vi "Sub Super Duper_6_26a_PD.vi"(0 "VISA resource name":refnum<visa-resource-name>="GPIB0::17::INSTR", 1 "Sample Properties:":T5 {"Date Created" format="%<%Y/%m/%d>T"}, 2 "TRF Cluster":T6={"Step 4"=-38.0, "# of Loops"=1.0, "Transfer 2"=FALSE, "Start 4"=-2.0, "Total Points 2"=2, "Start 3"=40.0, "Stop 2"=-40.0, "Step 3"=-1.0, "Loop Step"=0.0, "Integration Time 3"=0, "Loop Wait"=0.0, "First Step"=0.0} {"Loop Wait" format="%<%H:%M:%S>t"; "Integration Time 3" scale=0.0..2.0; "Step 3" format="%.2f"; "Stop 2" format="%.2f"; "Start 3" format="%.2f"; "Start 4" format="%.2f"; "Step 4" format="%.2f"}, 3 "TSP Cluster":T7={"Transport"=FALSE, "Start 2"=0.0, "Stop 3"=-60.0, "Step 2"=-1.0, "Start"=0.0, "Step"=-10.0, "Total Points"=7, "Integration Time"=0} {"Integration Time" scale=0.0..2.0; "Step" format="%.2f"; "Start" format="%.2f"; "Step 2" format="%.2f"; "Stop 3" format="%.2f"; "Start 2" format="%.2f"}, 4 "Compliance Cluster":T2={"Var1 sweep settings"={"sweep spacing (linear: 0)"=0, "sweep mode"=FALSE, "compliance (V)"=100.0, "compliance (A)"=0.001}, "Var1 sweep settings 2"={"sweep spacing (linear: 0)"=0, "sweep mode"=FALSE, "compliance (V)"=100.0, "compliance (A)"=0.001}, "Var2 step settings 2"={"compliance (A)"=0.001, "compliance (V)"=100.0}, "Var2 step settings"={"compliance (A)"=0.001, "compliance (V)"=100.0}} {"Var2 step settings"."compliance (V)" format="%.2f"; "Var2 step settings"."compliance (A)" format="%^.2e"; "Var2 step settings 2"."compliance (V)" format="%.2f"; "Var2 step settings 2"."compliance (A)" format="%^.2e"; "Var1 sweep settings 2"."compliance (A)" format="%^.2e"; "Var1 sweep settings 2"."compliance (V)" format="%.2f"; "Var1 sweep settings 2"."sweep spacing (linear: 0)" items=["linear", "log 10", "log 25", "log 50"]; "Var1 sweep settings"."compliance (A)" format="%^.2e"; "Var1 sweep settings"."compliance (V)" format="%.2f"; "Var1 sweep settings"."sweep spacing (linear: 0)" items=["linear", "log 10", "log 25", "log 50"]}, 5 "error in":errorcluster, 6 "Saved Folder:":path=path "C:/1DATA/2011", 7 "Wait Cluster":T1 {"Wait Time (s)" format="%.1g"; "Wait Countdown" format="%<%H:%M:%S%1u>t"}, 9 "Stop \nCountdown":bool) -> (8 "Status Indicator":bool, 14 "VISA resource name out":refnum<visa-resource-name>, 15 "TRF Path":path, 16 "TSP Path":path, 17 "Graph Cluster":T3, 18 "Char Cluster":T4, 19 "error out":errorcluster)   [LabVIEW 2011]
uses:
  <vilib>/Platform/TimedLoop/XDataNode/timing_clust.ctl
  <vilib>/Platform/TimedLoop/XDataNode/nitl_modes.ctl
  <vilib>/Platform/TimedLoop/XDataNode/wakeup.ctl
  <vilib>/Platform/TimedLoop/XDataNode/XDataNode.xnode
  <vilib>/Platform/TimedLoop/XDataNode/XDNodeRunTimeDep.lvlib
panel:
  in  "Transport Temp":cluster{"trace":dbl[], "trace":dbl[]}(graph)
  in  "Transfer Temp":cluster{dbl[], "trace":dbl[]}[](graph) caption="Transfer"
  out "graphic display":cluster{"trace":dbl[], "trace":dbl[]}(graph)
  # "Vg Sweep"
  # "Vd Step"
  # "Loops and Integration Time"
  # "Device Characteristics"
  # "Sample Properties:"
  # "%"
  # "nm"
  # "Device Properties:"
  # "um"
  # "um"
  # "Vg Step"
  # "Vd Step"
  # "Integration Time"
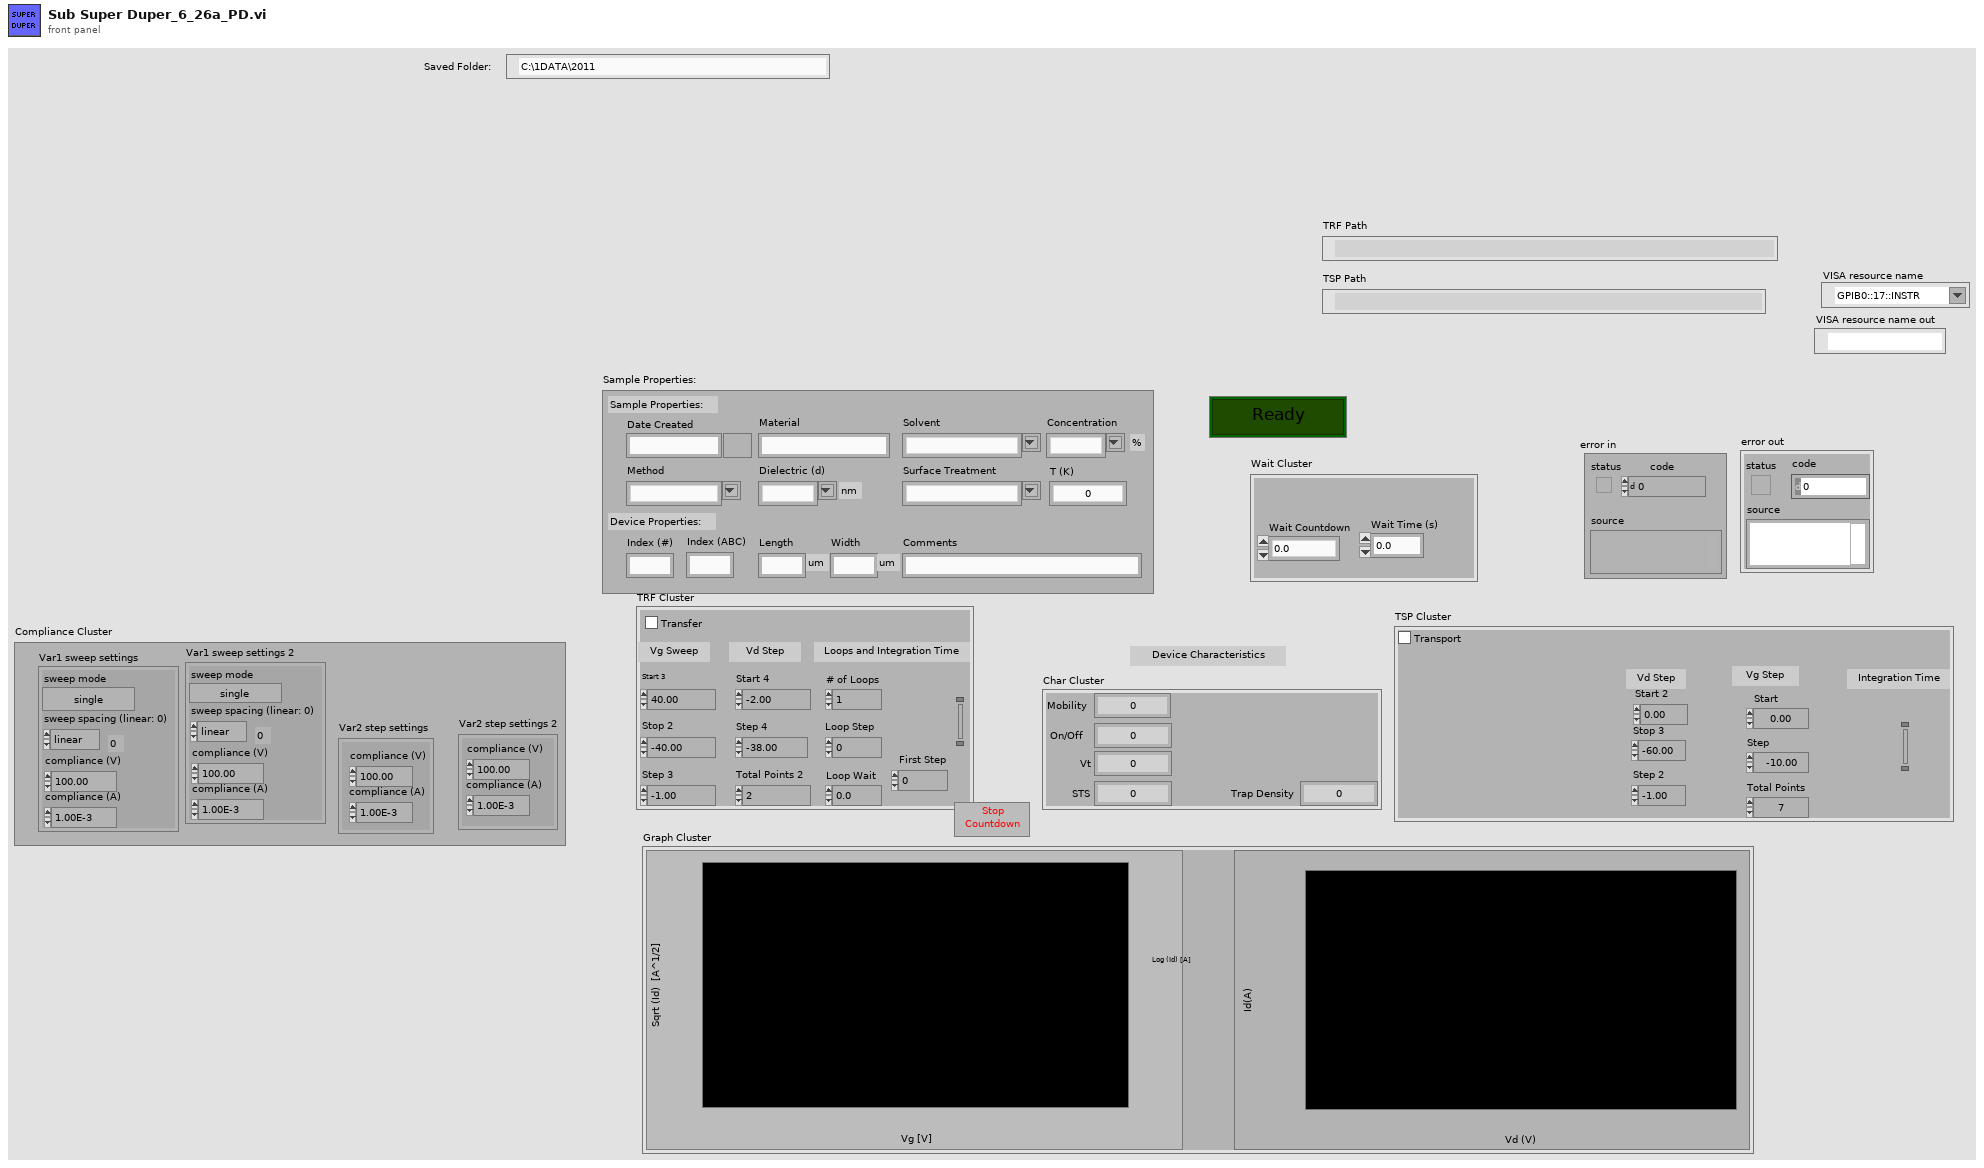
[diagram p1: front panel]
types:
  T1 = cluster{"Wait Countdown":dbl, "Wait Time (s)":dbl}
  T2 = cluster{"Var1 sweep settings":cluster{"sweep spacing (linear: 0)":u16, "sweep mode":bool, "compliance (V)":dbl, "compliance (A)":dbl}, "Var1 sweep settings 2":cluster{"sweep spacing (linear: 0)":u16, "sweep mode":bool, "compliance (V)":dbl, "compliance (A)":dbl}, "Var2 step settings 2":cluster{"compliance (A)":dbl, "compliance (V)":dbl}, "Var2 step settings":cluster{"compliance (A)":dbl, "compliance (V)":dbl}}
  T3 = cluster{"Transfer":cluster{dbl[], "trace":dbl[]}[], "Transport":cluster{"trace":dbl[], "trace":dbl[]}}
  T4 = cluster{"Mobility":dbl, "On/Off ":dbl, "Vt":dbl, "STS":dbl, "Trap Density":dbl}
  T5 = cluster{"Date Created":timestamp, "Material":string, "Solvent":string, "Concentration":string, "Method":string, "Dielectric (d)":string, "Index (#)":string, "Index (ABC)":string, "Length":string, "Width":string, "Surface Treatment":string, "Comments":string, "T (K)":dbl}
  T6 = cluster{"Step 4":dbl, "# of Loops":dbl, "Transfer 2":bool, "Start 4":dbl, "Total Points 2":u16, "Start 3":dbl, "Stop 2":dbl, "Step 3":dbl, "Loop Step":dbl, "Integration Time 3":u32, "Loop Wait":dbl, "First Step":dbl}
  T7 = cluster{"Transport":bool, "Start 2":dbl, "Stop 3":dbl, "Step 2":dbl, "Start":dbl, "Step":dbl, "Total Points":u16, "Integration Time":u32}
  T8 = typedef "XDNodeRunTimeDep.lvlib/timing_clust.ctl" = cluster{"Expected End [f-1]":u64, "Actual End [f-1]":u64, "Finished Late? [f-1]":bool, "Expected End [i-1]":u64, "Actual End [i-1]":u64, "Finished Late? [i-1]":bool, "Expected Start [i]":u64, "Actual Start [i]":u64, "Expected Start [f]":u64, "Actual Start [f]":u64, "Source Name":string, "Structure Name":string, "Period":i64, "Deadline":i64, "Offset":i64, "Start":i64, "Priority":i32, "Timeout":i32, "Mode":T9, "Wakeup Reason":T10, "Error":errorcluster, "Source Type":string, "Secondary Source Type":string, "Global End Time":u64, "Global Start Time":u64, "Frame Duration":u64, "Iteration Duration":u64, "Assigned CPU":i32, "I/O Scan Engine Mode":u32}
  T9 = typedef "XDNodeRunTimeDep.lvlib/nitl_modes.ctl" = enum32{"No Change", "Process missed periods, maintain original phase", "Discard missed periods, maintain original phase", "Process missed periods, ignore original phase", "Discard missed periods, ignore original phase"}
  T10 = typedef "XDNodeRunTimeDep.lvlib/wakeup.ctl" = enum32{"Normal", "Aborted", "Asynchronous wakeup", "Timing source error", "Timed loop error", "Timeout"}
  T11 = cluster{"sweep spacing (linear: 0)":u16, "sweep mode":bool, "compliance (V)":dbl, "compliance (A)":dbl}
  T12 = cluster{"compliance (A)":dbl, "compliance (V)":dbl}
  T13 = cluster{"Start 3":dbl, "Stop 2":dbl, "Step 3":dbl, "sweep spacing (linear: 0)":u16, "sweep mode":bool, "compliance (V)":dbl, "compliance (A)":dbl}
  T14 = cluster{"compliance (A)":dbl, "compliance (V)":dbl, "Start 4":dbl, "Total Points 2":u16, dbl}
  T15 = cluster{dbl, "# of Loops":dbl, "Transfer 2":bool, "Start 4":dbl, "Total Points 2":u16, "Start 3":dbl, "Stop 2":dbl, "Step 3":dbl, "Loop Step":dbl, "Integration Time 3":u32, "Loop Wait":dbl, "First Step":dbl}
  T16 = cluster{"Mobility":dbl, "On/Off Current":dbl, "Vt":dbl, "Trap Density":dbl, "STS":dbl}
  T17 = cluster{"Start 2":dbl, "Stop 3":dbl, "Step 2":dbl, "sweep spacing (linear: 0)":u16, "sweep mode":bool, "compliance (V)":dbl, "compliance (A)":dbl}
  T18 = cluster{"compliance (A)":dbl, "compliance (V)":dbl, "Start":dbl, "Total Points":u16, "Step":dbl}
  T19 = cluster{"Transfer Temp":cluster{dbl[], "trace":dbl[]}[], "Transport Temp":cluster{"trace":dbl[], "trace":dbl[]}}
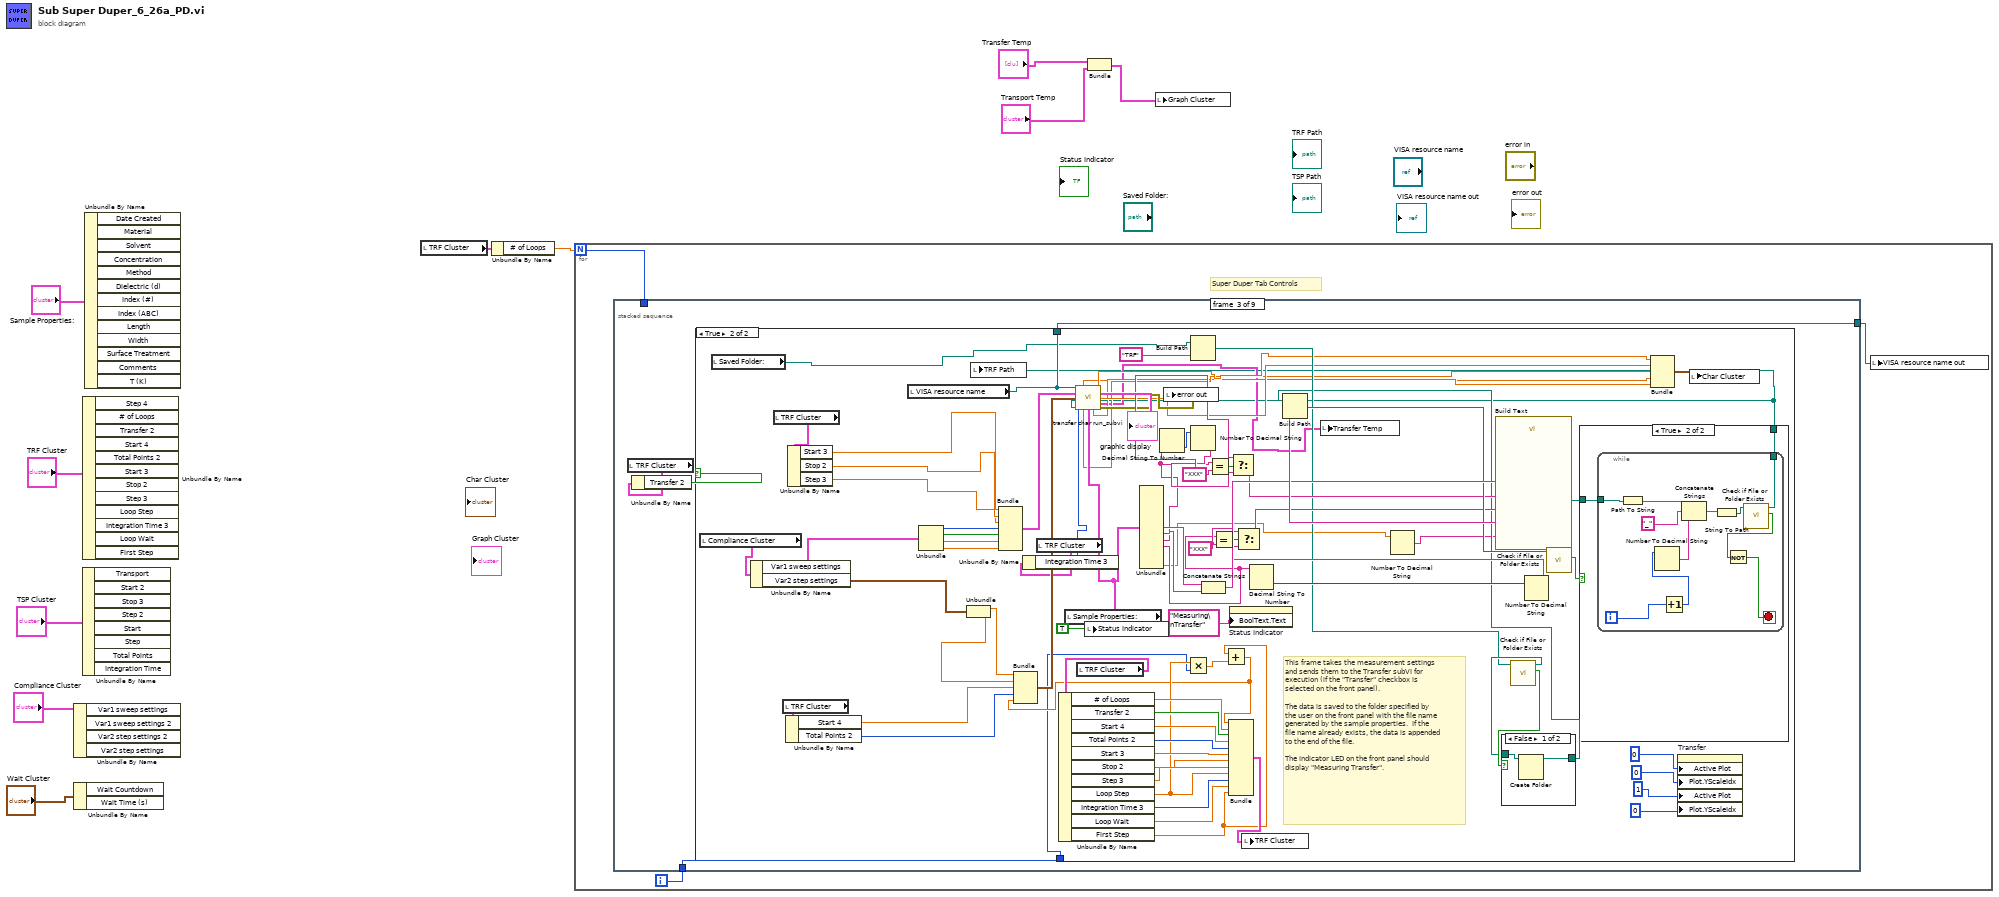
[diagram p0: block diagram]
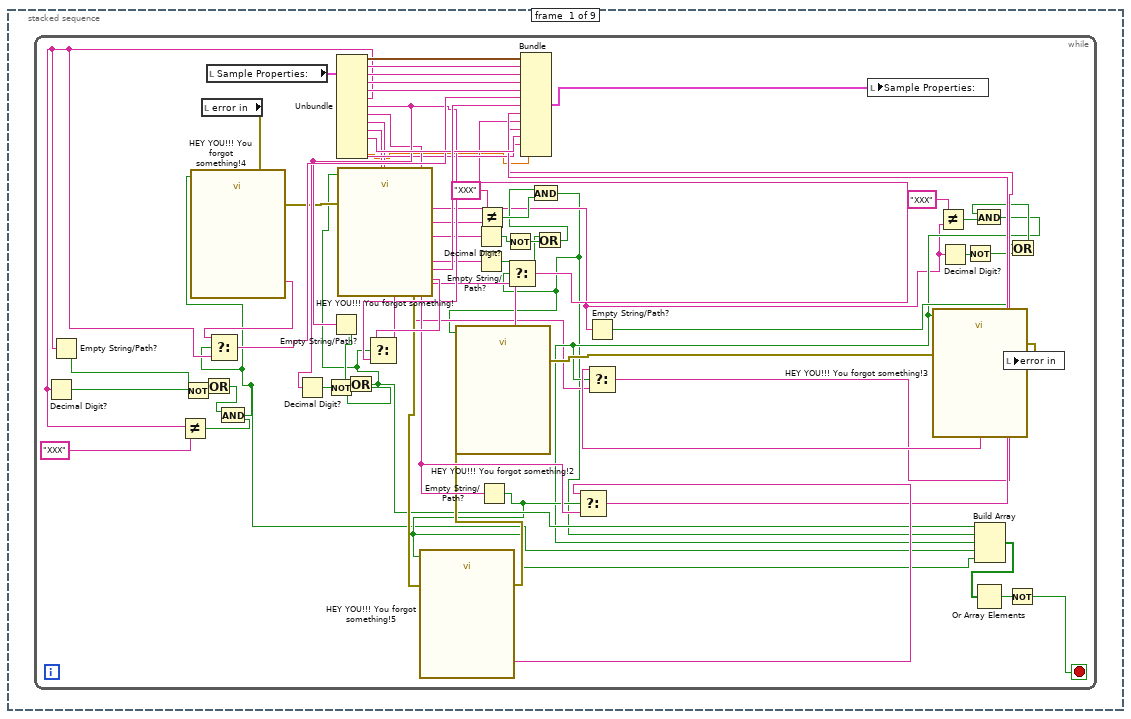
[diagram p2: hidden frame]
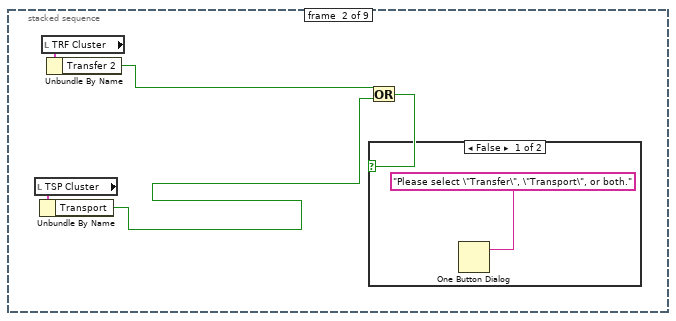
[diagram p3: hidden frame]
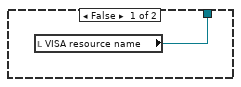
[diagram p5: hidden frame]
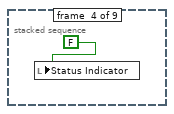
[diagram p8: hidden frame]
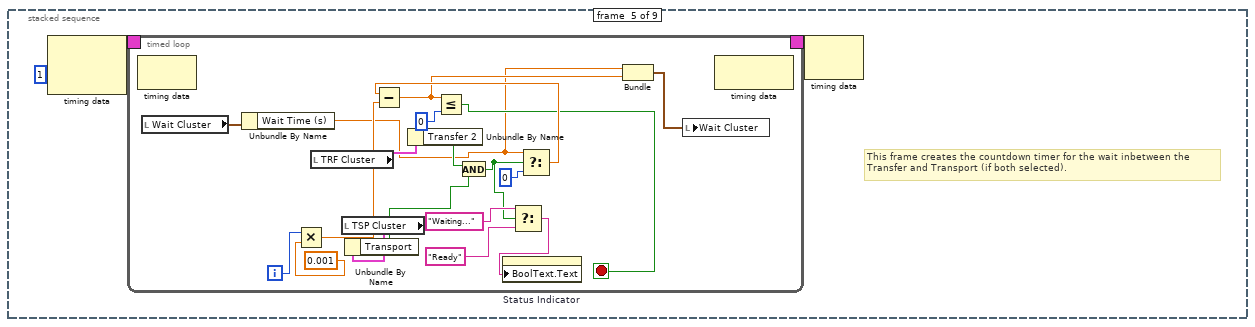
[diagram p9: hidden frame]
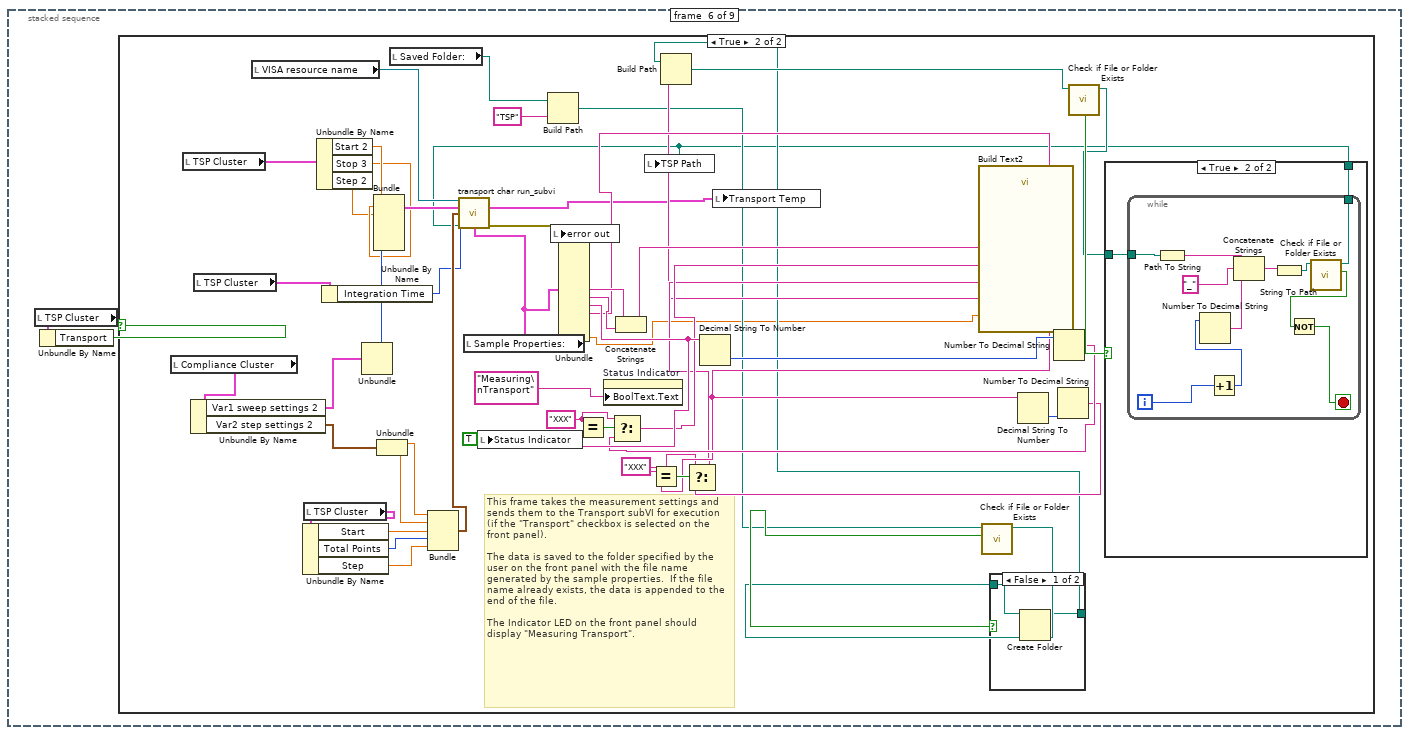
[diagram p10: hidden frame]
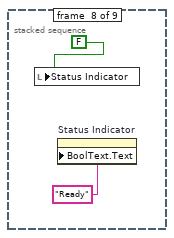
[diagram p15: hidden frame]
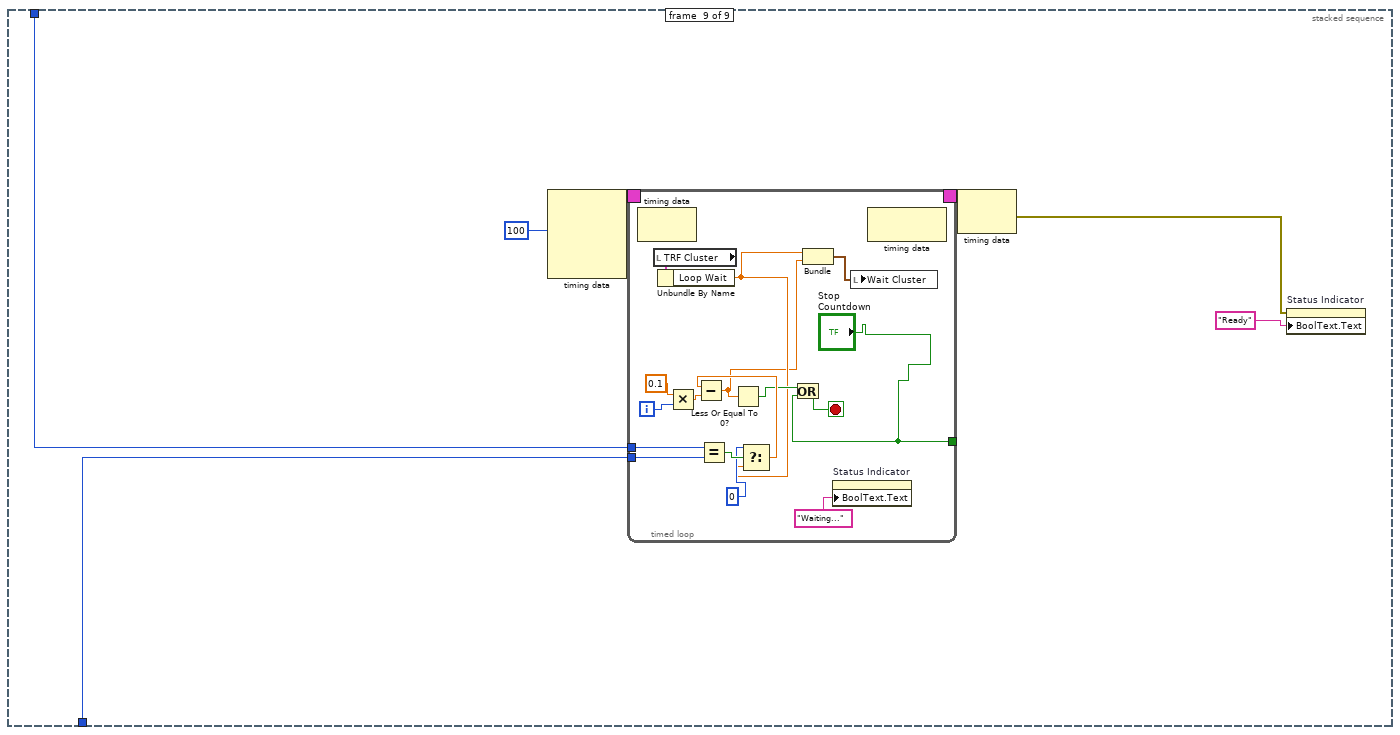
[diagram p16: hidden frame]
diagram:
  n1 = Unbundle By Name("Compliance Cluster") -> ()  [unwired: 4 out]
  n2 = Unbundle By Name("Wait Cluster") -> ()  [unwired: 2 out]
  n3 = Unbundle By Name("TSP Cluster") -> ()  [unwired: 8 out]
  n4 = Unbundle By Name("TRF Cluster") -> ()  [unwired: 12 out]
  n5 = Unbundle By Name("Sample Properties:") -> ()  [unwired: 13 out]
  n6 = local read "TRF Cluster"() -> (w10:T6)
  n7 = Unbundle By Name(w10) -> ("# of Loops"=w9:dbl)
  n8 = for {
    N: w9 -> [w12]
    i -> [w13]
    # "Super Duper Tab Controls"
    n9 = stacked-sequence {
      tunnel: w13 -> [_ _ w83 _ _ _ _ _ w288]
      tunnel: w12 -> [_ _ _ _ _ _ _ _ w287]
      tunnel: [_ _ w80 _ _ _ _ _ _] -> w11
      frame #0 {
        n10 = while {
          stop <- w39 stop-if-true
          n11 = local read "error in"() -> (w45:errorcluster)
          n12 = local read "Sample Properties:"() -> (w68:T5)
          n13 = Unbundle(w68) -> ("Date Created"=w69:timestamp, "Material"=w70:string, "Solvent"=w71:string, "Concentration"=w72:string, "Method"=w73:string, "Dielectric (d)"=w28:string, "Index (#)"=w58:string, "Index (ABC)"=w55:string, "Length"=w23:string, "Width"=w16:string, "Surface Treatment"=w61:string, "Comments"=w53:string, "T (K)"=w14:dbl)
          n14 = Decimal Digit?(1:w28) -> (0:w36:bool)
          n15 = Empty String/Path?(string/path=w28) -> (empty?=w30:bool)
          n16 = Not Equal?(x=w28, y="XXX") -> (x != y?=w27:bool)
          n17 = Not(x=w36) -> (.not. x?=w33:bool)
          n18 = Or(x=w30, y=w33) -> (x .or. y?=w26:bool)
          n19 = And(x=w26, y=w27) -> (x .and. y?=w25:bool)
          n20 = call "HEY YOU!!! You forgot something!4"("Enable"=w25, "error in (no error)"=w45) -> ("Dielectric (d)"=w60:string, "error out"=w44:errorcluster)  [unwired: 15 in, 1 out]
          n21 = Select(t=w60, s=w25, f=w28) -> (s? t:f=w59:string)
          n22 = Decimal Digit?(1:w58) -> (0:w49:bool)
          n23 = Not(x=w49) -> (.not. x?=w48:bool)
          n24 = Empty String/Path?(string/path=w58) -> (empty?=w57:bool)
          n25 = Or(x=w57, y=w48) -> (x .or. y?=w43:bool)
          n26 = call "HEY YOU!!! You forgot something!"("Enable"=w43, "error in (no error)"=w44) -> ("Index (#)"=w67:string, "error out"=w47:errorcluster)  [unwired: 15 in, 1 out]
          n27 = Select(t=w67, s=w43, f=w58) -> (s? t:f=w64:string)
          n28 = Decimal Digit?(1:w23) -> (0:w38:bool)
          n29 = Empty String/Path?(string/path=w23) -> (empty?=w32:bool)
          n30 = Not Equal?(x="XXX", y=w23) -> (x != y?=w22:bool)
          n31 = Empty String/Path?(string/path=w55) -> (empty?=w42:bool)
          n32 = call "HEY YOU!!! You forgot something!5"("Enable"=w42, "error in (no error)"=w47) -> ("Index (ABC)"=w56:string, "error out"=w46:errorcluster)  [unwired: 15 in, 1 out]
          n33 = Not(x=w38) -> (.not. x?=w35:bool)
          n34 = Or(x=w32, y=w35) -> (x .or. y?=w21:bool)
          n35 = And(x=w21, y=w22) -> (x .and. y?=w15:bool)
          n36 = call "HEY YOU!!! You forgot something!2"("Enable"=w15, "error in (no error)"=w46) -> ("Length"=w66:string, "error out"=w63:errorcluster)  [unwired: 15 in, 1 out]
          n37 = Select(t=w66, s=w15, f=w23) -> (s? t:f=w52:string)
          n38 = Select(t=w56, s=w42, f=w55) -> (s? t:f=w54:string)
          n39 = Empty String/Path?(string/path=w16) -> (empty?=w31:bool)
          n40 = Not Equal?(x="XXX", y=w16) -> (x != y?=w20:bool)
          n41 = Decimal Digit?(1:w16) -> (0:w37:bool)
          n42 = Not(x=w37) -> (.not. x?=w34:bool)
          n43 = Or(x=w31, y=w34) -> (x .or. y?=w19:bool)
          n44 = And(x=w19, y=w20) -> (x .and. y?=w18:bool)
          n45 = call "HEY YOU!!! You forgot something!3"("Enable"=w18, "error in (no error)"=w63) -> ("Width"=w65:string, "error out"=w62:errorcluster)  [unwired: 15 in, 1 out]
          n46 = Select(t=w65, s=w18, f=w16) -> (s? t:f=w51:string)
          n47 = Bundle("Date Created"=w69, "Material"=w70, "Solvent"=w71, "Concentration"=w72, "Method"=w73, "Dielectric (d)"=w59, "Index (#)"=w64, "Index (ABC)"=w54, "Length"=w52, "Width"=w51, "Surface Treatment"=w61, "Comments"=w53, "T (K)"=w14) -> (w50:T5)  [unwired: 1 in]
          n48 = local write "Sample Properties:"(w50) -> ()
          n49 = Build Array(w43, w15, w18, w25, w42) -> (w41:bool[])
          n50 = Or Array Elements(Boolean array=w41) -> (logical OR=w40:bool)
          n51 = local write "error in"(w62) -> ()
          n52 = Not(x=w40) -> (.not. x?=w39:bool)
        }
      }
      frame #1 {
        n53 = local read "TSP Cluster"() -> (w75:T7)
        n54 = Unbundle By Name(w75) -> ("Transport"=w74:bool)
        n55 = local read "TRF Cluster"() -> (w77:T6)
        n56 = Unbundle By Name(w77) -> ("Transfer 2"=w76:bool)
        n57 = Or(x=w76, y=w74) -> (x .or. y?=w78:bool)
        n58 = case shown="False" w78 {
          frame False {
            n59 = One Button Dialog(message="Please select \"Transfer\", \"Transport\", or both.") -> ()  [unwired: 1 in, 1 out]
          }
          frame True {
          }
        }
      }
      frame #2 {
        n60 = local read "TRF Cluster"() -> (w81:T6)
        n61 = Unbundle By Name(w81) -> ("Transfer 2"=w82:bool)
        n62 = case shown="True" w82 {
          tunnel: w83 -> [_ w86]
          tunnel: [w84 w97] -> w80
          frame False {
            n63 = local read "VISA resource name"() -> (w84:refnum<visa-resource-name>)
          }
          frame True {
            w140 = "XXX"
            w144 = "XXX"
            # "This frame takes the measurement settings and sends them to the Transfer subVI for execution (if the \"Transfer\" checkbox is selected on the front panel).\n\nThe data is saved to the folder specified by the user on the front panel with the file name generated by the sample properties.  If the file name already exists, the data is appended to the end of the file.\n\nThe Indicator LED on the front panel should display \"Measuring Transfer\"."
            n64 = local read "Compliance Cluster"() -> (w94:T2)
            n65 = local read "Saved Folder:"() -> (w96:path)
            n66 = Unbundle By Name(w94) -> ("Var1 sweep settings"=w92:T11, "Var2 step settings"=w93:T12)
            n67 = local read "TRF Cluster"() -> (w121:T6)
            n68 = local read "TRF Cluster"() -> (w124:T6)
            n69 = Unbundle By Name(w124) -> ("Start 4"=w123:dbl, "Total Points 2"=w122:u16)
            n70 = Unbundle By Name(w121) -> ("Start 3"=w120:dbl, "Stop 2"=w119:dbl, "Step 3"=w118:dbl)
            n71 = local read "VISA resource name"() -> (w97:refnum<visa-resource-name>)
            n72 = Unbundle(w92) -> ("sweep spacing (linear: 0)"=w165:u16, "sweep mode"=w164:bool, "compliance (V)"=w163:dbl, "compliance (A)"=w162:dbl)
            n73 = Unbundle(w93) -> ("compliance (A)"=w160:dbl, "compliance (V)"=w159:dbl)
            n74 = Bundle("Start 3"=w120, "Stop 2"=w119, "Step 3"=w118, "sweep spacing (linear: 0)"=w165, "sweep mode"=w164, "compliance (V)"=w163, "compliance (A)"=w162) -> (w161:T13)  [unwired: 1 in]
            n75 = local read "TRF Cluster"() -> (w116:T6)
            n76 = Unbundle By Name(w116) -> ("Integration Time 3"=w117:u32)
            n77 = local read "Sample Properties:"() -> (w126:T5)
            n78 = local read "TRF Cluster"() -> (w106:T6)
            n79 = Unbundle By Name(w106) -> ("# of Loops"=w107:dbl, "Transfer 2"=w108:bool, "Start 4"=w109:dbl, "Total Points 2"=w110:u16, "Start 3"=w111:dbl, "Stop 2"=w112:dbl, "Step 3"=w113:dbl, "Loop Step"=w88:dbl, "Integration Time 3"=w114:u32, "Loop Wait"=w115:dbl, "First Step"=w85:dbl)
            n80 = local write "Status Indicator"(TRUE) -> ()
            n81 = Unbundle(w126) -> ("Index (#)"=w153:string, "Index (ABC)"=w152:string, "Length"=w136:string, "Width"=w139:string, "T (K)"=w91:dbl)  [unwired: 8 out]
            n82 = Decimal String To Number(string=w136) -> (number=w147:i32)  [unwired: 2 in, 1 out]
            n83 = Multiply(x=w88, y=w86) -> (x*y=w89:dbl)
            n84 = Build Path(base path=w96, name or relative path="TRF") -> (appended path=w132:path)
            n85 = Number To Decimal String(number=w147) -> (decimal integer string=w143:string)  [unwired: 1 in]
            n86 = Concatenate Strings(w153, w152) -> (w151:string)
            n87 = Equal?(x=w136, y=w144) -> (x = y?=w145:bool)
            n88 = Equal?(x=w139, y=w140) -> (x = y?=w141:bool)
            n89 = Add(x=w85, y=w89) -> (x+y=w87:dbl)
            n90 = Bundle("compliance (A)"=w160, "compliance (V)"=w159, "Start 4"=w123, "Total Points 2"=w122, w87) -> (w158:T14)  [unwired: 1 in]
            n91 = Bundle ("Bundle Again")(w87, "# of Loops"=w107, "Transfer 2"=w108, "Start 4"=w109, "Total Points 2"=w110, "Start 3"=w111, "Stop 2"=w112, "Step 3"=w113, "Loop Step"=w88, "Integration Time 3"=w114, "Loop Wait"=w115, "First Step"=w85) -> (w105:T15)  [unwired: 1 in]
            n92 = property on="Status Indicator" class="Bool (strict)"("BoolText.Text"="Measuring\nTransfer") -> ()  [unwired: 2 in, 2 out]
            n93 = Select(t=w144, s=w145, f=w143) -> (s? t:f=w142:string)
            n94 = local write "TRF Cluster"(w105) -> ()
            n95 = Decimal String To Number(string=w139) -> (number=w146:i32)  [unwired: 2 in, 1 out]
            n96 = Number To Decimal String(number=w91) -> (decimal integer string=w90:string)  [unwired: 1 in]
            n97 = call <vilib>:"Check if File or Folder Exists.vi"("path"=w132) -> ("file or folder exists?"=w134:bool, "dup path"=w133:path)  [unwired: 8 in, 1 out]
            n98 = case shown="False" w134 {
              tunnel: w133 -> [w167 w168]
              tunnel: [w166 w168] -> w131
              frame False {
                n99 = Create Folder(path (use dialog)=w167) -> (created path=w166:path)  [unwired: 2 in, 2 out]
              }
              frame True {
              }
            }
            n100 = Number To Decimal String(number=w146) -> (decimal integer string=w138:string)  [unwired: 1 in]
            n101 = Select(t=w140, s=w141, f=w138) -> (s? t:f=w137:string)
            n102 = call "Build Text"("T"=w90, "Index"=w151, "Length"=w142, "Width"=w137) -> ("Result"=w157:string)  [unwired: 10 in, 1 out]
            n103 = Build Path(base path=w131, name or relative path=w157) -> (appended path=w149:path)
            n104 = call <vilib>:"Check if File or Folder Exists.vi"("path"=w149) -> ("file or folder exists?"=w150:bool, "dup path"=w148:path)  [unwired: 8 in, 1 out]
            n105 = case shown="True" w150 {
              tunnel: w148 -> [w169 w171]
              tunnel: [w169 w170] -> w95
              frame False {
              }
              frame True {
                n106 = while {
                  tunnel: w171 -> [w173]
                  tunnel: [w172] -> w170
                  i -> [w175]
                  stop <- w176 stop-if-true
                  n107 = Path To String(path=w173) -> (string=w182:string)
                  n108 = Increment(x=w175) -> (x+1=w174:i32)
                  n109 = Number To Decimal String(number=w174) -> (decimal integer string=w180:string)  [unwired: 1 in]
                  n110 = Concatenate Strings(w182, "_", w180) -> (w179:string)
                  n111 = String To Path(string=w179) -> (path=w178:path)
                  n112 = call <vilib>:"Check if File or Folder Exists.vi"("path"=w178) -> ("file or folder exists?"=w177:bool, "dup path"=w172:path)  [unwired: 8 in, 1 out]
                  n113 = Not(x=w177) -> (.not. x?=w176:bool)
                }
              }
            }
            n114 = local write "TRF Path"(w95) -> ()
            n115 = call "transfer char run_subvi.vi"("VISA session"=w97, "Var1 sweep settings"=w161, "Var2 step settings"=w158, "integration time"=w117, "Path"=w95, "Sample Properties:"=w126) -> ("Trap Density"=w99:dbl, "Mobility"=w103:dbl, "graphic display"=→"graphic display":cluster{"trace":dbl[], "trace":dbl[]}, "On/Off Current"=w102:dbl, "XY Graph"=w98:cluster{dbl[], "trace":dbl[]}[], "Vt"=w101:dbl, "STS"=w100:dbl, "error?"=w125:errorcluster)  [unwired: 2 in]
            n116 = local write "error out"(w125) -> ()
            n117 = local write "Transfer Temp"(w98) -> ()
            n118 = Bundle("Mobility"=w103, "On/Off Current"=w102, "Vt"=w101, "Trap Density"=w99, "STS"=w100) -> (w104:T16)  [unwired: 1 in]
            n119 = property on="Transfer" class="XYGraph (strict)"("Active Plot"=0, "Plot.YScaleIdx"=0, "Active Plot"=1, "Plot.YScaleIdx"=0) -> ()  [unwired: 2 in, 2 out]
            n120 = local write "Char Cluster"(w104) -> ()
          }
        }
      }
      frame #3 {
        n121 = local write "Status Indicator"(FALSE) -> ()
      }
      frame #4 {
        # "This frame creates the countdown timer for the wait inbetween the\nTransfer and Transport (if both selected)."
        n122 = node-c288(1) -> (w186:T8)  [unwired: 1 in]
        n123 = timed-loop {
          timing: w186 -> [_]
          timing-out: [_] -> w185
          i -> [w197]
          stop <- w198 stop-if-true
          n124 = node-c288() -> ()  [unwired: 1 in, 1 out]
          n125 = local read "Wait Cluster"() -> (w190:T1)
          n126 = Unbundle By Name(w190) -> ("Wait Time (s)"=w188:dbl)
          n127 = Multiply(x=w197, y=0.001) -> (x*y=w195:dbl)
          n128 = local read "TRF Cluster"() -> (w191:T6)
          n129 = local read "TSP Cluster"() -> (w192:T7)
          n130 = Unbundle By Name(w192) -> ("Transport"=w193:bool)
          n131 = Unbundle By Name(w191) -> ("Transfer 2"=w194:bool)
          n132 = And(x=w194, y=w193) -> (x .and. y?=w202:bool)
          n133 = Select(t="Waiting...", s=w202, f="Ready") -> (s? t:f=w204:string)
          n134 = property on="Status Indicator" class="Bool (strict)"("BoolText.Text"=w204) -> ()  [unwired: 2 in, 2 out]
          n135 = Select(t=w188, s=w202, f=0) -> (s? t:f=w200:dbl)
          n136 = Subtract(x=w200, y=w195) -> (x-y=w189:dbl)
          n137 = Less Or Equal?(x=w189, y=0) -> (x <= y?=w198:bool)
          n138 = Bundle("Wait Time (s)"=w188, w189) -> (w187:cluster{"Wait Time (s)":dbl, dbl})  [unwired: 1 in]
          n139 = local write "Wait Cluster"(w187) -> ()
          n140 = node-c288() -> ()  [unwired: 1 in, 1 out]
        }
        n141 = node-c288(w185) -> ()  [unwired: 1 out]
      }
      frame #5 {
        n142 = local read "TSP Cluster"() -> (w213:T7)
        n143 = Unbundle By Name(w213) -> ("Transport"=w212:bool)
        n144 = case shown="True" w212 {
          frame False {
          }
          frame True {
            w240 = "XXX"
            w244 = "XXX"
            # "This frame takes the measurement settings and sends them to the Transport subVI for execution (if the \"Transport\" checkbox is selected on the front panel).\n\nThe data is saved to the folder specified by the user on the front panel with the file name generated by the sample properties.  If the file name already exists, the data is appended to the end of the file.\n\nThe Indicator LED on the front panel should display \"Measuring Transport\"."
            n145 = local read "Compliance Cluster"() -> (w218:T2)
            n146 = local read "TSP Cluster"() -> (w231:T7)
            n147 = Unbundle By Name(w218) -> ("Var1 sweep settings 2"=w217:T11, "Var2 step settings 2"=w216:T12)
            n148 = local read "TSP Cluster"() -> (w224:T7)
            n149 = local read "VISA resource name"() -> (w220:refnum<visa-resource-name>)
            n150 = local read "TSP Cluster"() -> (w222:T7)
            n151 = Unbundle By Name(w222) -> ("Start"=w227:dbl, "Total Points"=w226:u16, "Step"=w225:dbl)
            n152 = Unbundle By Name(w231) -> ("Start 2"=w230:dbl, "Stop 3"=w229:dbl, "Step 2"=w228:dbl)
            n153 = Unbundle By Name(w224) -> ("Integration Time"=w223:u32)
            n154 = Unbundle(w217) -> ("sweep spacing (linear: 0)"=w267:u16, "sweep mode"=w266:bool, "compliance (V)"=w265:dbl, "compliance (A)"=w264:dbl)
            n155 = Bundle("Start 2"=w230, "Stop 3"=w229, "Step 2"=w228, "sweep spacing (linear: 0)"=w267, "sweep mode"=w266, "compliance (V)"=w265, "compliance (A)"=w264) -> (w263:T17)  [unwired: 1 in]
            n156 = Unbundle(w216) -> ("compliance (A)"=w262:dbl, "compliance (V)"=w261:dbl)
            n157 = local read "Saved Folder:"() -> (w219:path)
            n158 = Bundle("compliance (A)"=w262, "compliance (V)"=w261, "Start"=w227, "Total Points"=w226, "Step"=w225) -> (w260:T18)  [unwired: 1 in]
            n159 = local read "Sample Properties:"() -> (w256:T5)
            n160 = local write "Status Indicator"(TRUE) -> ()
            n161 = Build Path(base path=w219, name or relative path="TSP") -> (appended path=w233:path)
            n162 = Unbundle(w256) -> ("Index (#)"=w255:string, "Index (ABC)"=w254:string, "Length"=w245:string, "Width"=w241:string, "T (K)"=w214:dbl)  [unwired: 8 out]
            n163 = Equal?(x=w244, y=w245) -> (x = y?=w246:bool)
            n164 = property on="Status Indicator" class="Bool (strict)"("BoolText.Text"="Measuring\nTransport") -> ()  [unwired: 2 in, 2 out]
            n165 = Concatenate Strings(w255, w254) -> (w253:string)
            n166 = Equal?(x=w240, y=w241) -> (x = y?=w249:bool)
            n167 = Decimal String To Number(string=w245) -> (number=w248:i32)  [unwired: 2 in, 1 out]
            n168 = call <vilib>:"Check if File or Folder Exists.vi"("path"=w233) -> ("file or folder exists?"=w235:bool, "dup path"=w234:path)  [unwired: 8 in, 1 out]
            n169 = case shown="False" w235 {
              tunnel: w234 -> [w269 w270]
              tunnel: [w268 w270] -> w232
              frame False {
                n170 = Create Folder(path (use dialog)=w269) -> (created path=w268:path)  [unwired: 2 in, 2 out]
              }
              frame True {
              }
            }
            n171 = Decimal String To Number(string=w241) -> (number=w247:i32)  [unwired: 2 in, 1 out]
            n172 = Number To Decimal String(number=w248) -> (decimal integer string=w243:string)  [unwired: 1 in]
            n173 = Select(t=w244, s=w246, f=w243) -> (s? t:f=w242:string)
            n174 = Number To Decimal String(number=w247) -> (decimal integer string=w239:string)  [unwired: 1 in]
            n175 = Select(t=w240, s=w249, f=w239) -> (s? t:f=w238:string)
            n176 = call "Build Text2"("T"=w214, "Index"=w253, "Length"=w242, "Width"=w238) -> ("Result"=w237:string)  [unwired: 10 in, 1 out]
            n177 = Build Path(base path=w232, name or relative path=w237) -> (appended path=w250:path)
            n178 = call <vilib>:"Check if File or Folder Exists.vi"("path"=w250) -> ("file or folder exists?"=w252:bool, "dup path"=w251:path)  [unwired: 8 in, 1 out]
            n179 = case shown="True" w252 {
              tunnel: w251 -> [w271 w273]
              tunnel: [w271 w272] -> w215
              frame False {
              }
              frame True {
                n180 = while {
                  tunnel: w273 -> [w275]
                  tunnel: [w274] -> w272
                  i -> [w277]
                  stop <- w278 stop-if-true
                  n181 = Path To String(path=w275) -> (string=w284:string)
                  n182 = Increment(x=w277) -> (x+1=w276:i32)
                  n183 = Number To Decimal String(number=w276) -> (decimal integer string=w282:string)  [unwired: 1 in]
                  n184 = Concatenate Strings(w284, "_", w282) -> (w281:string)
                  n185 = String To Path(string=w281) -> (path=w280:path)
                  n186 = call <vilib>:"Check if File or Folder Exists.vi"("path"=w280) -> ("file or folder exists?"=w279:bool, "dup path"=w274:path)  [unwired: 8 in, 1 out]
                  n187 = Not(x=w279) -> (.not. x?=w278:bool)
                }
              }
            }
            n188 = call "transport char run_subvi.vi"("VISA session"=w220, "Var1 sweep settings"=w263, "Var2 step settings"=w260, "integration time"=w223, "Path"=w215, "Sample Properties:"=w256) -> ("graphic display"=w221:cluster{"trace":dbl[], "trace":dbl[]}, "error?"=w259:errorcluster)  [unwired: 8 in]
            n189 = local write "error out"(w259) -> ()
            n190 = local write "TSP Path"(w215) -> ()
            n191 = local write "Transport Temp"(w221) -> ()
          }
        }
      }
      frame #6 {
      }
      frame #7 {
        n192 = local write "Status Indicator"(FALSE) -> ()
        n193 = property on="Status Indicator" class="Bool (strict)"("BoolText.Text"="Ready") -> ()  [unwired: 2 in, 2 out]
      }
      frame #8 {
        n194 = node-c288(100) -> (w293:T8)  [unwired: 3 in]
        n195 = timed-loop {
          timing: w293 -> [_]
          timing-out: [_] -> w292
          tunnel: w288 -> [w304]
          tunnel: w287 -> [w303]
          tunnel: ["Stop \nCountdown"] -> _
          i -> [w309]
          stop <- w299 stop-if-true
          n196 = node-c288() -> ()  [unwired: 1 in, 1 out]
          n197 = local read "TRF Cluster"() -> (w298:T6)
          n198 = Unbundle By Name(w298) -> ("Loop Wait"=w296:dbl)
          n199 = Multiply(x=0.1, y=w309) -> (x*y=w307:dbl)
          n200 = Equal?(x=w303, y=w304) -> (x = y?=w305:bool)
          n201 = Select(t=0, s=w305, f=w296) -> (s? t:f=w301:dbl)
          n202 = Subtract(x=w301, y=w307) -> (x-y=w295:dbl)
          n203 = Less Or Equal To 0?(x=w295) -> (x <= 0?=w300:bool)
          n204 = Or(x=w300, y="Stop \nCountdown") -> (x .or. y?=w299:bool)
          n205 = Bundle("Loop Wait"=w296, w295) -> (w297:cluster{"Loop Wait":dbl, dbl})  [unwired: 1 in]
          n206 = property on="Status Indicator" class="Bool (strict)"("BoolText.Text"="Waiting...") -> ()  [unwired: 2 in, 2 out]
          n207 = local write "Wait Cluster"(w297) -> ()
          n208 = node-c288() -> ()  [unwired: 1 in, 1 out]
        }
        n209 = node-c288(w292) -> (w289:errorcluster)
        n210 = property on="Status Indicator" class="Bool (strict)"(error in=w289, "BoolText.Text"="Ready") -> ()  [unwired: 1 in, 2 out]
      }
    }
    n211 = local write "VISA resource name out"(w11) -> ()
  }
  n212 = Bundle("Transfer Temp"="Transfer Temp", "Transport Temp"="Transport Temp") -> (w6:T19)  [unwired: 1 in]
  n213 = local write "Graph Cluster"(w6) -> ()
